vi "Handle Message.vi"(8 "error in":errorcluster, 10 "Message":T1, 11 "Vision Server in":refnum<class "Vision Server.lvclass">) -> (0 "error out":errorcluster, 3 "Vision Server out":refnum<class "Vision Server.lvclass">)   [LabVIEW 2016, in "Vision Server.lvclass"]
uses:
  Vision Server.lvclass
  typedef/Message Type.ctl
  Vision Server.lvclass/Vision Server.ctl
  typedef/Target Message JSON.ctl
  typedef/Target Vector.ctl
  typedef/Target Message Processed.ctl
  typedef/Sensor Message JSON.ctl
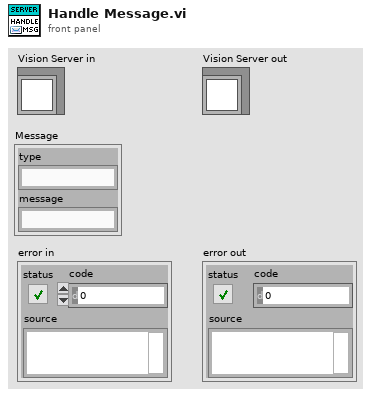
[diagram p1: front panel]
types:
  T1 = typedef "Vision Server.lvclass/Message Type.ctl" = cluster{"type":string, "message":string}
  T2 = typedef "Vision Server.lvclass/Target Message Processed.ctl" = cluster{"timestamp":u32, "targets":T3[]}
  T3 = typedef "Vision Server.lvclass/Target Vector.ctl" = cluster{"y":dbl, "z":dbl}
  T4 = typedef "Vision Server.lvclass/Target Message JSON.ctl" = cluster{"capturedAgoMs":i32, "targets":T3[]}
  T5 = typedef "Vision Server.lvclass/Sensor Message JSON.ctl" = cluster{"azimuth":dbl, "pitch":dbl, "roll":dbl}
  T6 = typedef "Vision Server.lvclass/Target Listener Queue.ctl" = refnum<queue>
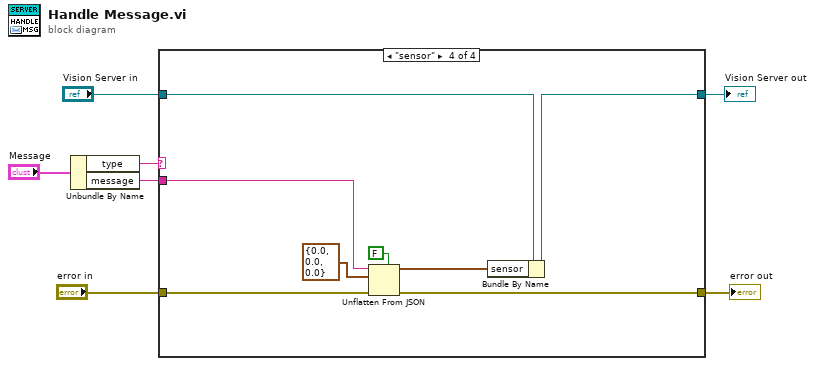
[diagram p0: block diagram]
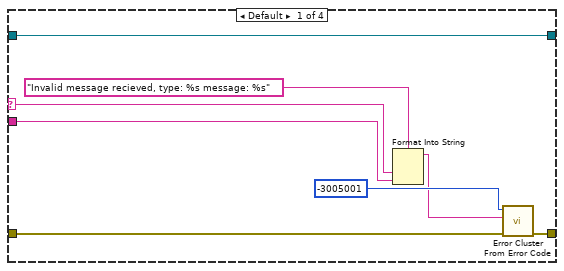
[diagram p2: hidden frame]
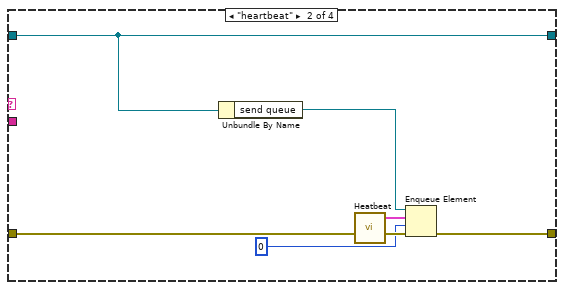
[diagram p3: hidden frame]
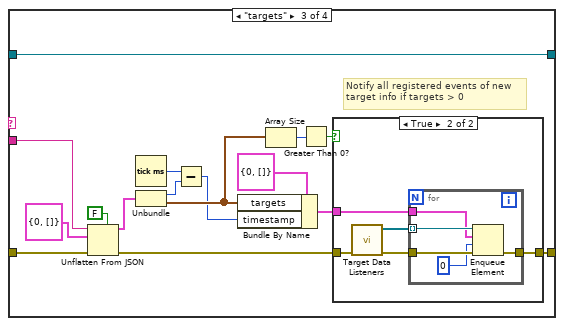
[diagram p4: hidden frame]
diagram:
  n1 = Unbundle By Name("Message") -> ("type"=w2:string, "message"=w1:string)
  n2 = case shown="\"sensor\"" w2 {
    selector: w2 -> [w12 _ _ _]
    tunnel: "error in" -> [w15 w19 w33 w53]
    tunnel: [w13 w18 w31 w51] -> w5
    tunnel: "Vision Server in" -> [w14 w21 w37 w56]
    tunnel: [w14 w21 w37 w50] -> w7
    tunnel: w1 -> [w11 _ w36 w55]
    frame Default {
      n3 = Format Into String(format string="Invalid message recieved, type: %s message: %s" ("error message (\"\")"), w12, w11) -> (resulting string=w8:string)  [unwired: 2 in, 1 out]
      n4 = call <vilib>:"Error Cluster From Error Code.vi"("error in (no error)"=w15, "error message (\"\")"=w8, "error code (0)"=-3005001) -> ("error out"=w13:errorcluster)  [unwired: 6 in]
    }
    frame "heartbeat" {
      n5 = Unbundle By Name(w21) -> ("send queue"=w20:refnum<queue>)
      n6 = call "Heatbeat.vi"() -> ("camera mode vision"=w17:T1)  [unwired: 2 in]
      n7 = Enqueue Element(queue=w20, element=w17, timeout in ms (-1)=0, error in (no error)=w19) -> (error out=w18:errorcluster)  [unwired: 2 out]
    }
    frame "targets" {
      # "Notify all registered events of new\ntarget info if targets > 0"
      n8 = Unflatten From JSON(enable LabVIEW extensions? (T)=FALSE, JSON string=w36, type and defaults=T4 {"capturedAgoMs"=0, "targets"=[]}, error in (no error)=w33) -> (value=w26:T4, error out=w32:errorcluster)  [unwired: 3 in]
      n9 = Tick Count (ms)() -> (millisecond timer value=w24:u32)
      n10 = Unbundle(w26) -> ("capturedAgoMs"=w23:i32, "targets"=w25:T3[])
      n11 = Subtract(x=w24, y=w23) -> (x-y=w22:u32)
      n12 = Bundle By Name(cluster=T2 {"timestamp"=0, "targets"=[]} ("Target Msg"), "targets"=w25, "timestamp"=w22) -> (w27:T2)
      n13 = Array Size(array=w25) -> (size(s)=w29:i32)
      n14 = Greater Than 0?(x=w29) -> (x > 0?=w30:bool)
      n15 = case shown="True" w30 {
        tunnel: w32 -> [w38 w39]
        tunnel: w27 -> [_ w41]
        tunnel: [w38 w40] -> w31
        frame False {
          # "0 targets found"
        }
        frame True {
          n16 = call "Target Data Listeners.vi"("error in"=w39) -> ("error out"=w43:errorcluster, "Listeners"=w42:T6[])  [unwired: 9 in]
          n17 = for {
            tunnel: w43 -> [w47]
            tunnel: w42 -> [w48] mode=indexing
            tunnel: w41 -> [w46]
            tunnel: [w44] -> w40
            n18 = Enqueue Element(queue=w48, element=w46, timeout in ms (-1)=0, error in (no error)=w47) -> (error out=w44:errorcluster)  [unwired: 2 out]
          }
        }
      }
    }
    frame "sensor" {
      n19 = Unflatten From JSON(enable LabVIEW extensions? (T)=FALSE, JSON string=w55, type and defaults=T5 {"azimuth"=0.0, "pitch"=0.0, "roll"=0.0} ("Sensor Msg"), error in (no error)=w53) -> (value=w49:T5, error out=w51:errorcluster)  [unwired: 3 in]
      n20 = Bundle By Name(cluster=w56, "sensor"=w49) -> (w50:refnum<class "Vision Server.lvclass">)
    }
  }
  "Vision Server out" <- w7
  "error out" <- w5
